vi "PreScanCheck.vi"(11 "Input":string="34,45,89") -> (1 "error":bool, 2 "error":errorcluster, 3 "concatenated error":string)   [LabVIEW 2014]
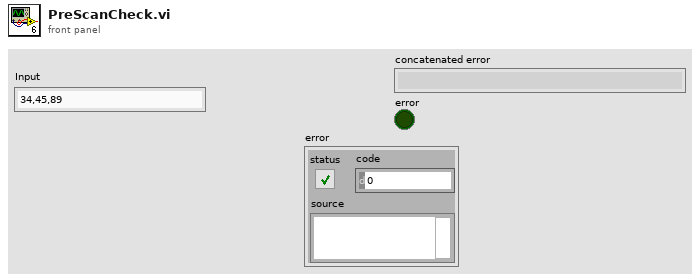
[diagram p1: front panel]
types:
  T1 = enum16{"pixel", "position", "size", "dip", "bias", "timing"}
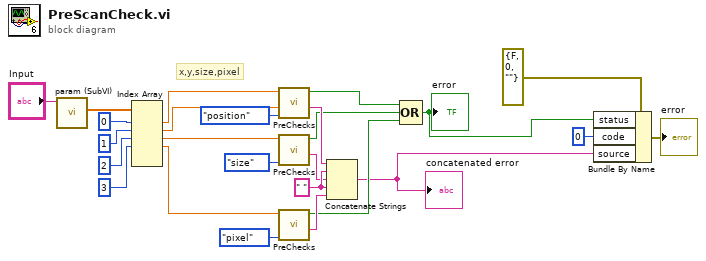
[diagram p0: block diagram]
diagram:
  w14 = " " ("string")
  # "x,y,size,pixel"
  n1 = call <userlib>:"param (SubVI).vi"("Input"="Input") -> ("parm"=w25:dbl[])  [unwired: 8 in, 2 out]
  n2 = Index Array(array=w25, index #1=0 ("index"), index #2=1 ("index"), index #3=2 ("index"), index #4=3 ("index")) -> (element #1=w19:dbl, element #2=w18:dbl, element #3=w16:dbl, element #4=w17:dbl)  [unwired: 2 in, 2 out]
  n3 = call "PreChecks.vi"("type"=T1."position", "Y"=w18, "X"=w19) -> ("message"=w15:string, "Error"=w11:bool)  [unwired: 7 in]
  n4 = call "PreChecks.vi"("type"=T1."size", "X"=w16) -> ("message"=w13:string, "Error"=w10:bool)  [unwired: 8 in]
  n5 = call "PreChecks.vi"("type"=T1."pixel", "X"=w17) -> ("message"=w12:string, "Error"=w9:bool)  [unwired: 8 in]
  n6 = Concatenate Strings(w15, w14, w13, w14, w12) -> (w6:string)
  "concatenated error" <- w6
  n7 = Compound Arithmetic op=OR(w11, w10, w9) -> (w7:bool)
  "error" <- w7
  n8 = Bundle By Name(cluster=errorcluster {"status"=FALSE, "code"=0, "source"=""} ("error in (no error)"), "status"=w7, "code"=0, "source"=w6) -> (→"error":errorcluster)
